vi "validate.vi"(8 "error in":errorcluster, 11 "Tagbus PID Module configuration in":refnum<class "Tagbus PID Module configuration.lvclass">) -> (0 "error out":errorcluster, 3 "Tagbus PID Module configuration out":refnum<class "Tagbus PID Module configuration.lvclass">)   [LabVIEW 2014, in "Tagbus PID Module configuration.lvclass"]
doc: "This function performs validation of the configuration. This function should be safe to call at any point and should not rely on anything in the runtime environment."
uses:
  Tagbus PID Module configuration.lvclass
  <vilib>/NI/Tag Bus Module Framework/module configuration/TBM module configuration.lvclass
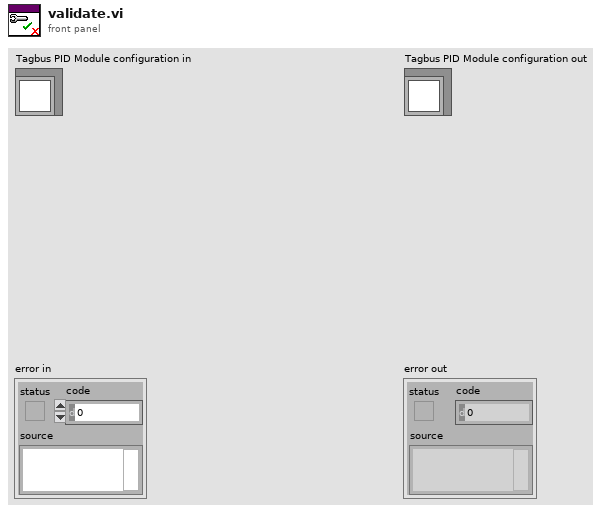
[diagram p1: front panel]
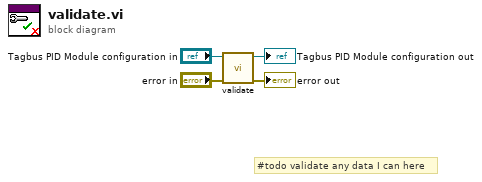
[diagram p0: block diagram]
diagram:
  # "#todo validate any data I can here"
  n1 = call-parent "validate.vi"("error in"="error in", "configuration in"="Tagbus PID Module configuration in") -> ("error out"=→"error out":errorcluster, "configuration out"=→"Tagbus PID Module configuration out":refnum<class "Tagbus PID Module configuration.lvclass">)  [unwired: 8 in]
